vi "Swerve Math.vi"(9 "Yaw":dbl, 10 "Rot. Point Y":dbl, 11 "Rot. Point X":dbl) -> (3 "Swerve Math Ouput":dbl[](array[numeric]))   [LabVIEW 2018]
uses:
  Drive Train Global.vi
  Robot Information/Robot Information Global.vi
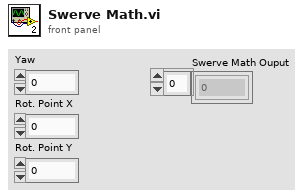
[diagram p1: front panel]
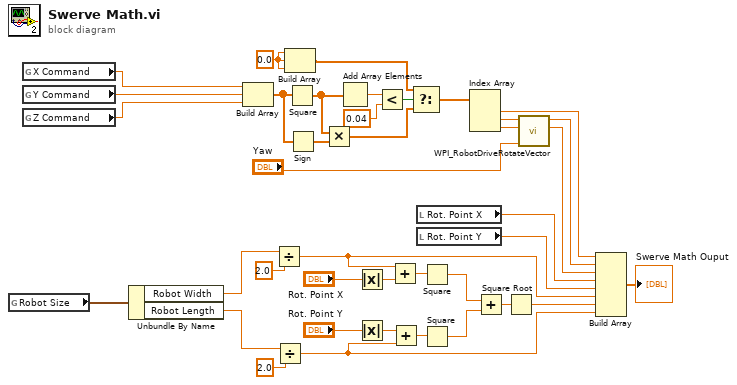
[diagram p0: block diagram]
diagram:
  w8 = 0.0 ("element")
  n1 = global read "Robot Information Global.vi" "Robot Size"() -> (w15:cluster{"Robot Width":dbl, "Robot Length":dbl})
  n2 = global read "Drive Train Global.vi" "X Command"() -> (w16:dbl)
  n3 = global read "Drive Train Global.vi" "Y Command"() -> (w2:dbl)
  n4 = global read "Drive Train Global.vi" "Z Command"() -> (w17:dbl)
  n5 = Unbundle By Name(w15) -> ("Robot Width"=w13:dbl, "Robot Length"=w14:dbl)
  n6 = Build Array(w16, w2, w17) -> (w4:dbl[])
  n7 = Divide(x=w13, y=2.0) -> (x/y=w25:dbl)
  n8 = Divide(x=w14, y=2.0) -> (x/y=w23:dbl)
  n9 = Build Array(w8, w8, w8) -> (w9:dbl[])
  n10 = Square(x=w4) -> (x^2=w6:dbl[])
  n11 = Sign(1:w4) -> (0:w7:dbl[])
  n12 = Multiply(x=w6, y=w7) -> (x*y=w5:dbl[])
  n13 = Add Array Elements(numeric array=w6) -> (sum=w12:dbl)
  n14 = Absolute Value(x="Rot. Point X") -> (abs(x)=w39:dbl)
  n15 = Absolute Value(x="Rot. Point Y") -> (abs(x)=w37:dbl)
  n16 = Less?(x=w12, y=0.04 ("x")) -> (x < y?=w10:bool)
  n17 = Add(x=w25, y=w39) -> (x+y=w38:dbl)
  n18 = Add(x=w37, y=w23) -> (x+y=w36:dbl)
  n19 = Select(t=w9, s=w10, f=w5) -> (s? t:f=w21:dbl[])
  n20 = local read "Rot. Point X"() -> (w27:dbl)
  n21 = local read "Rot. Point Y"() -> (w26:dbl)
  n22 = Square(x=w38) -> (x^2=w34:dbl)
  n23 = Square(x=w36) -> (x^2=w35:dbl)
  n24 = Index Array(array=w21) -> (element #1=w19:dbl, element #2=w22:dbl, element #3=w28:dbl)  [unwired: 3 in]
  n25 = Add(x=w34, y=w35) -> (x+y=w33:dbl)
  n26 = Square Root(x=w33) -> (sqrt(x)=w24:dbl)
  n27 = call <vilib>:"WPI_RobotDriveRotateVector.vi"("Angle"="Yaw", "X"=w28, "Y"=w22) -> ("X'"=w20:dbl, "Y'"=w18:dbl)  [unwired: 7 out]
  n28 = Build Array(w19, w18, w20, w27, w26, w25, w24, w23) -> (→"Swerve Math Ouput":dbl[])
